vi "AttriClusterTemp.vi"() -> ()   [LabVIEW 2012]
uses:
  GraphAttriCluster.ctl
  GraphStates.ctl
  WaveGraphX.xctl
panel:
  in  "属性簇":T1={"曲线条数"=0, "曲线属性簇数组"=[], "文本属性簇数组"=[], "信息属性簇"={"图例"=FALSE, "信息_统计量"=FALSE, "信息_统计量_有效值"=FALSE, "信息_统计量_最大值"=FALSE, "信息_统计量_最小值"=FALSE, "信息_统计量_峰峰值"=FALSE, "信息_统计量_均值"=FALSE, "信息_统计量_方差"=FALSE, "信息_统计量_所有通道"=FALSE, "光标列表"=0, "数量"=1.0, "排列"=0, "格式"=0, "精度"=3.0}} {"信息属性簇"."格式" items=["十进制", "科学值"]; "信息属性簇"."排列" items=["幅值"]; "信息属性簇"."光标列表" items=["单光标", "双光标", "峰值光标"]; "曲线属性簇数组"."曲线_填充基线" items=["无", "零", "负无穷大", "正无穷大"]; "曲线属性簇数组"."曲线_线条宽度" items=["0", "1", "2", "3", "4", "5"]; "曲线属性簇数组"."曲线_线条样式" items=["实线", "粗虚线", "细虚线", "点划线", "双点划线"]}
  in  "信息属性簇":T2={"图例"=FALSE, "信息_统计量"=FALSE, "信息_统计量_有效值"=FALSE, "信息_统计量_最大值"=FALSE, "信息_统计量_最小值"=FALSE, "信息_统计量_峰峰值"=FALSE, "信息_统计量_均值"=FALSE, "信息_统计量_方差"=FALSE, "信息_统计量_所有通道"=FALSE, "光标列表"=0, "数量"=1.0, "排列"=0, "格式"=0, "精度"=3.0} {"格式" items=["十进制", "科学值"]; "排列" items=["幅值"]; "光标列表" items=["单光标", "双光标", "峰值光标"]}
  in  "文本属性簇":T3
  in  "曲线属性簇":T4 {"曲线_填充基线" items=["无", "零", "负无穷大", "正无穷大"]; "曲线_线条宽度" items=["0", "1", "2", "3", "4", "5"]; "曲线_线条样式" items=["实线", "粗虚线", "细虚线", "点划线", "双点划线"]}
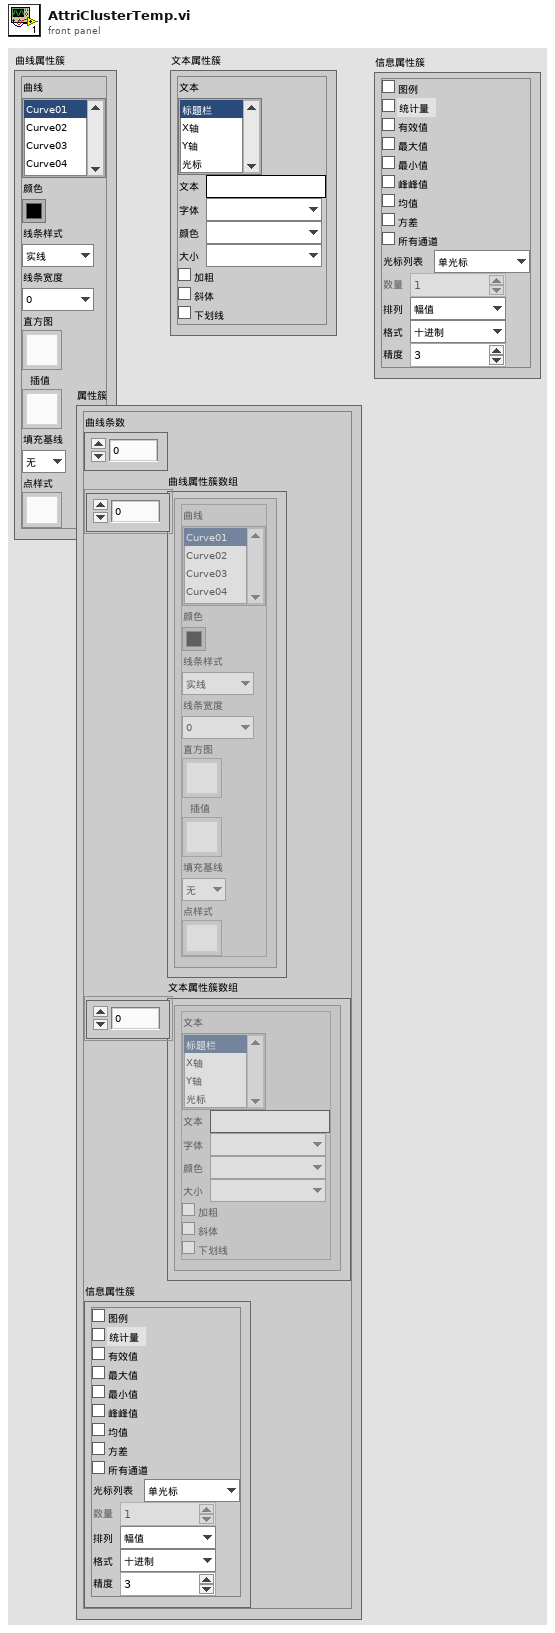
[diagram p1: front panel]
types:
  T1 = typedef "WaveGraphX.xctl/GraphStates.ctl" = cluster{"曲线条数":u8, "曲线属性簇数组":cluster{"曲线_曲线":i32, "曲线_颜色":u32, "曲线_线条样式":u16, "曲线_线条宽度":u16, "曲线_直方图":u16, "曲线_插值":u16, "曲线_填充基线":u16, "曲线_点样式":u16}[], "文本属性簇数组":cluster{"文本_文本":i32, "文本":string, "字体":u16, "颜色":u16, "大小":u16, "加粗":bool, "斜体":bool, "下划线":bool}[], "信息属性簇":cluster{"图例":bool, "信息_统计量":bool, "信息_统计量_有效值":bool, "信息_统计量_最大值":bool, "信息_统计量_最小值":bool, "信息_统计量_峰峰值":bool, "信息_统计量_均值":bool, "信息_统计量_方差":bool, "信息_统计量_所有通道":bool, "光标列表":u16, "数量":dbl, "排列":u16, "格式":u16, "精度":dbl}}
  T2 = cluster{"图例":bool, "信息_统计量":bool, "信息_统计量_有效值":bool, "信息_统计量_最大值":bool, "信息_统计量_最小值":bool, "信息_统计量_峰峰值":bool, "信息_统计量_均值":bool, "信息_统计量_方差":bool, "信息_统计量_所有通道":bool, "光标列表":u16, "数量":dbl, "排列":u16, "格式":u16, "精度":dbl}
  T3 = cluster{"文本_文本":i32, "文本":string, "字体":u16, "颜色":u16, "大小":u16, "加粗":bool, "斜体":bool, "下划线":bool}
  T4 = typedef "WaveGraphX.xctl/GraphAttriCluster.ctl" = cluster{"曲线_曲线":i32, "曲线_颜色":u32, "曲线_线条样式":u16, "曲线_线条宽度":u16, "曲线_直方图":u16, "曲线_插值":u16, "曲线_填充基线":u16, "曲线_点样式":u16}
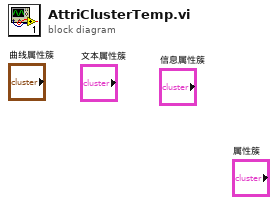
[diagram p0: block diagram]
diagram:
